vi "DrawPlayerNumber.vi"(8 "error in (no error)":errorcluster, 10 "Accessors:Singleplayer":bool, 11 "Game in":refnum<class "Game.lvclass">) -> (0 "error out":errorcluster)   [LabVIEW 2019, in "RT_Game.lvlib" / "GameMenu.lvclass"]
uses:
  GameMenu.lvclass
  Game/Game.lvclass
  Game/Coordinate.ctl
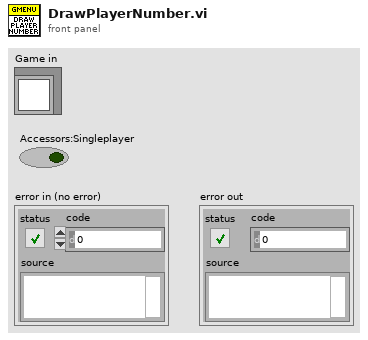
[diagram p1: front panel]
types:
  T1 = typedef "RT_Game.lvlib/Game.lvclass/Coordinate.ctl" = cluster{"x":dbl, "y":dbl}
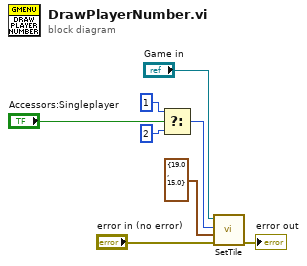
[diagram p0: block diagram]
diagram:
  n1 = Select(t=u32 1 ("Numeric"), s="Accessors:Singleplayer", f=u32 2 ("Numeric")) -> (s? t:f=w5:u32)
  n2 = call "SetTile.vi"("error in (no error)"="error in (no error)", "Coordinates"=T1 {"x"=19.0, "y"=15.0} ("Position"), "TileNumber"=w5, "Game in"="Game in") -> ("error out"=→"error out":errorcluster)  [unwired: 6 in, 1 out]
